vi "S4GUI.vi"() -> ()   [LabVIEW 2018] (continued)
        n871 = call-dynamic "Write State Machine.vi"("error in (no error)"=w1797, "State Machine.lvclass"=w1799, "Device in"=w1801) -> ("error out"=w1782:errorcluster, "Device out"=w1778:refnum<class "Channel.lvclass">)  [unwired: 7 in]
        n872 = call "Write section_name.vi"("error in (no error)"=w1782, "section_name"="CCD_ACS1", "Channel in"=w1778) -> ("error out"=w1783:errorcluster, "Channel out"=w1777:refnum<class "Channel.lvclass">)  [unwired: 7 in]
        n873 = call-dynamic "save config.vi"("error in (no error)"=w1783, "file config"="lastsaved.cfg", "Channel in"=w1777) -> ("error out"=w1781:errorcluster, "Channel out"=w1776:refnum<class "Channel.lvclass">)  [unwired: 7 in]
        n874 = call-dynamic "Write Channel.vi"("error in (no error)"=w1781, "Channel.lvclass"=w1776, "Acquisition in"=w1803) -> ("error out"=w1795:errorcluster, "Acquisition out"=w1794:refnum<class "Acquisition.lvclass">)  [unwired: 7 in]
        n875 = call-dynamic "Write AcquisitionA.vi"("error in (no error)"=w1795, "Acquisition.lvclass"=w1794, "S4ACS_GUI in"=w1805) -> ("error out"=w1793:errorcluster, "S4ACS_GUI out"=w1784:refnum<class "S4GUI.lvclass">)  [unwired: 7 in]
      }
      event "Load Button": Value Change {
        n876 = event-data() -> ()  [unwired: 1 in, 6 out]
        n877 = call <vilib>:"Application Directory.vi"() -> ("Application Directory"=w1819:path)
        n878 = call "File Dialog"("start path"=w1819, "prompt"="Select file...", "button label"="Open", "default name"="lastsaved.cfg", "error in"=w1813, "pattern (all files)"="*.cfg") -> ("selected path"=w1811:path, "cancelled"=w1814:bool, "error out"=→"error out 2":errorcluster)  [unwired: 6 in, 1 out]
        "selected path" <- w1811
        n879 = Path To String(path=w1811) -> (string=w1810:string)
        n880 = Match Pattern(string=w1810, regular expression="SPARC4_GUI\\") -> (after substring=w1808:string)  [unwired: 1 in, 3 out]
        n881 = case shown="False" w1814 {
          tunnel: w1822 -> [w1931 w1933]
          tunnel: [w1847 w1933] -> w1821
          tunnel: [w1845 w1932] -> w1820
          tunnel: w1813 -> [w1844 w1932]
          tunnel: w1808 -> [w1843 _]
          frame False {
            n882 = call-dynamic "Read AcquisitionA.vi"("error in (no error)"=w1844, "S4ACS_GUI in"=w1931) -> ("error out"=w1927:errorcluster, "Acquisition.lvclass"=w1929:refnum<class "Acquisition.lvclass">, "S4ACS_GUI out"=w1930:refnum<class "S4GUI.lvclass">)  [unwired: 7 in]
            n883 = call-dynamic "Read Channel.vi"("error in (no error)"=w1927, "Acquisition in"=w1929) -> ("error out"=w1914:errorcluster, "Channel.lvclass"=w1916:refnum<class "Channel.lvclass">, "Acquisition out"=w1928:refnum<class "Acquisition.lvclass">)  [unwired: 7 in]
            n884 = call "Write section_name.vi"("error in (no error)"=w1914, "section_name"="CCD_ACS1", "Channel in"=w1916) -> ("error out"=w1913:errorcluster, "Channel out"=w1915:refnum<class "Channel.lvclass">)  [unwired: 7 in]
            n885 = call-dynamic "load config.vi"("error in (no error)"=w1913, "cfg file name"=w1843, "Channel in"=w1915) -> ("error out"=w1839:errorcluster, "Channel out"=w1841:refnum<class "Channel.lvclass">)  [unwired: 7 in]
            n886 = call-dynamic "save config.vi"("error in (no error)"=w1839, "file config"="lastsaved.cfg", "Channel in"=w1841) -> ("error out"=w1842:errorcluster, "Channel out"=w1840:refnum<class "Channel.lvclass">)  [unwired: 7 in]
            n887 = call-dynamic "Read State Machine.vi"("error in (no error)"=w1842, "Device in"=w1840) -> ("error out"=w1923:errorcluster, "State Machine.lvclass"=w1925:refnum<class "State Machine.lvclass">, "Device out"=w1926:refnum<class "Channel.lvclass">)  [unwired: 7 in]
            n888 = call-dynamic "Write State.vi"("error in (no error)"=w1923, "State"=60, "State Machine in"=w1925) -> ("error out"=w1922:errorcluster, "State Machine out"=w1924:refnum<class "State Machine.lvclass">)  [unwired: 7 in]
            n889 = call-dynamic "Write State Machine.vi"("error in (no error)"=w1922, "State Machine.lvclass"=w1924, "Device in"=w1926) -> ("error out"=w1919:errorcluster, "Device out"=w1920:refnum<class "Channel.lvclass">)  [unwired: 7 in]
            n890 = call-dynamic "Write Channel.vi"("error in (no error)"=w1919, "Channel.lvclass"=w1920, "Acquisition in"=w1928) -> ("error out"=w1918:errorcluster, "Acquisition out"=w1917:refnum<class "Acquisition.lvclass">)  [unwired: 7 in]
            n891 = call-dynamic "Write AcquisitionA.vi"("error in (no error)"=w1918, "Acquisition.lvclass"=w1917, "S4ACS_GUI in"=w1930) -> ("error out"=w1854:errorcluster, "S4ACS_GUI out"=w1853:refnum<class "S4GUI.lvclass">)  [unwired: 7 in]
            n892 = call "Read AcquisitionB.vi"("error in (no error)"=w1854, "S4ACS_GUI in"=w1853) -> ("error out"=w1896:errorcluster, "Acquisition.lvclass"=w1894:refnum<class "Acquisition.lvclass">, "S4ACS_GUI out"=w1893:refnum<class "S4GUI.lvclass">)  [unwired: 7 in]
            n893 = call-dynamic "Read Channel.vi"("error in (no error)"=w1896, "Acquisition in"=w1894) -> ("error out"=w1909:errorcluster, "Channel.lvclass"=w1907:refnum<class "Channel.lvclass">, "Acquisition out"=w1895:refnum<class "Acquisition.lvclass">)  [unwired: 7 in]
            n894 = call "Write section_name.vi"("error in (no error)"=w1909, "section_name"="CCD_ACS2", "Channel in"=w1907) -> ("error out"=w1910:errorcluster, "Channel out"=w1908:refnum<class "Channel.lvclass">)  [unwired: 7 in]
            n895 = call-dynamic "load config.vi"("error in (no error)"=w1910, "cfg file name"=w1843, "Channel in"=w1908) -> ("error out"=w1836:errorcluster, "Channel out"=w1834:refnum<class "Channel.lvclass">)  [unwired: 7 in]
            n896 = call-dynamic "save config.vi"("error in (no error)"=w1836, "file config"="lastsaved.cfg", "Channel in"=w1834) -> ("error out"=w1835:errorcluster, "Channel out"=w1833:refnum<class "Channel.lvclass">)  [unwired: 7 in]
            n897 = call-dynamic "Read State Machine.vi"("error in (no error)"=w1835, "Device in"=w1833) -> ("error out"=w1900:errorcluster, "State Machine.lvclass"=w1898:refnum<class "State Machine.lvclass">, "Device out"=w1897:refnum<class "Channel.lvclass">)  [unwired: 7 in]
            n898 = call-dynamic "Write State.vi"("error in (no error)"=w1900, "State"=60, "State Machine in"=w1898) -> ("error out"=w1901:errorcluster, "State Machine out"=w1899:refnum<class "State Machine.lvclass">)  [unwired: 7 in]
            n899 = call-dynamic "Write State Machine.vi"("error in (no error)"=w1901, "State Machine.lvclass"=w1899, "Device in"=w1897) -> ("error out"=w1904:errorcluster, "Device out"=w1903:refnum<class "Channel.lvclass">)  [unwired: 7 in]
            n900 = call-dynamic "Write Channel.vi"("error in (no error)"=w1904, "Channel.lvclass"=w1903, "Acquisition in"=w1895) -> ("error out"=w1905:errorcluster, "Acquisition out"=w1906:refnum<class "Acquisition.lvclass">)  [unwired: 7 in]
            n901 = call "Write AcquisitionB.vi"("error in (no error)"=w1905, "Acquisition.lvclass"=w1906, "S4ACS_GUI in"=w1893) -> ("error out"=w1852:errorcluster, "S4ACS_GUI out"=w1851:refnum<class "S4GUI.lvclass">)  [unwired: 7 in]
            n902 = call-dynamic "Read AcquisitionC.vi"("error in (no error)"=w1852, "S4ACS_GUI in"=w1851) -> ("error out"=w1889:errorcluster, "Acquisition.lvclass"=w1891:refnum<class "Acquisition.lvclass">, "S4ACS_GUI out"=w1892:refnum<class "S4GUI.lvclass">)  [unwired: 7 in]
            n903 = call-dynamic "Read Channel.vi"("error in (no error)"=w1889, "Acquisition in"=w1891) -> ("error out"=w1876:errorcluster, "Channel.lvclass"=w1878:refnum<class "Channel.lvclass">, "Acquisition out"=w1890:refnum<class "Acquisition.lvclass">)  [unwired: 7 in]
            n904 = call "Write section_name.vi"("error in (no error)"=w1876, "section_name"="CCD_ACS3", "Channel in"=w1878) -> ("error out"=w1875:errorcluster, "Channel out"=w1877:refnum<class "Channel.lvclass">)  [unwired: 7 in]
            n905 = call-dynamic "load config.vi"("error in (no error)"=w1875, "cfg file name"=w1843, "Channel in"=w1877) -> ("error out"=w1831:errorcluster, "Channel out"=w1829:refnum<class "Channel.lvclass">)  [unwired: 7 in]
            n906 = call-dynamic "save config.vi"("error in (no error)"=w1831, "file config"="lastsaved.cfg", "Channel in"=w1829) -> ("error out"=w1830:errorcluster, "Channel out"=w1828:refnum<class "Channel.lvclass">)  [unwired: 7 in]
            n907 = call-dynamic "Read State Machine.vi"("error in (no error)"=w1830, "Device in"=w1828) -> ("error out"=w1885:errorcluster, "State Machine.lvclass"=w1887:refnum<class "State Machine.lvclass">, "Device out"=w1888:refnum<class "Channel.lvclass">)  [unwired: 7 in]
            n908 = call-dynamic "Write State.vi"("error in (no error)"=w1885, "State"=60, "State Machine in"=w1887) -> ("error out"=w1884:errorcluster, "State Machine out"=w1886:refnum<class "State Machine.lvclass">)  [unwired: 7 in]
            n909 = call-dynamic "Write State Machine.vi"("error in (no error)"=w1884, "State Machine.lvclass"=w1886, "Device in"=w1888) -> ("error out"=w1881:errorcluster, "Device out"=w1882:refnum<class "Channel.lvclass">)  [unwired: 7 in]
            n910 = call-dynamic "Write Channel.vi"("error in (no error)"=w1881, "Channel.lvclass"=w1882, "Acquisition in"=w1890) -> ("error out"=w1880:errorcluster, "Acquisition out"=w1879:refnum<class "Acquisition.lvclass">)  [unwired: 7 in]
            n911 = call-dynamic "Write AcquisitionC.vi"("error in (no error)"=w1880, "Acquisition.lvclass"=w1879, "S4ACS_GUI in"=w1892) -> ("error out"=w1850:errorcluster, "S4ACS_GUI out"=w1849:refnum<class "S4GUI.lvclass">)  [unwired: 7 in]
            n912 = call-dynamic "Read AcquisitionD.vi"("error in (no error)"=w1850, "S4ACS_GUI in"=w1849) -> ("error out"=w1858:errorcluster, "Acquisition.lvclass"=w1856:refnum<class "Acquisition.lvclass">, "S4ACS_GUI out"=w1855:refnum<class "S4GUI.lvclass">)  [unwired: 7 in]
            n913 = call-dynamic "Read Channel.vi"("error in (no error)"=w1858, "Acquisition in"=w1856) -> ("error out"=w1871:errorcluster, "Channel.lvclass"=w1869:refnum<class "Channel.lvclass">, "Acquisition out"=w1857:refnum<class "Acquisition.lvclass">)  [unwired: 7 in]
            n914 = call "Write section_name.vi"("error in (no error)"=w1871, "section_name"="CCD_ACS4", "Channel in"=w1869) -> ("error out"=w1872:errorcluster, "Channel out"=w1870:refnum<class "Channel.lvclass">)  [unwired: 7 in]
            n915 = call-dynamic "load config.vi"("error in (no error)"=w1872, "cfg file name"=w1843, "Channel in"=w1870) -> ("error out"=w1827:errorcluster, "Channel out"=w1825:refnum<class "Channel.lvclass">)  [unwired: 7 in]
            n916 = call-dynamic "save config.vi"("error in (no error)"=w1827, "file config"="lastsaved.cfg", "Channel in"=w1825) -> ("error out"=w1826:errorcluster, "Channel out"=w1824:refnum<class "Channel.lvclass">)  [unwired: 7 in]
            n917 = call-dynamic "Read State Machine.vi"("error in (no error)"=w1826, "Device in"=w1824) -> ("error out"=w1862:errorcluster, "State Machine.lvclass"=w1860:refnum<class "State Machine.lvclass">, "Device out"=w1859:refnum<class "Channel.lvclass">)  [unwired: 7 in]
            n918 = call-dynamic "Write State.vi"("error in (no error)"=w1862, "State"=60, "State Machine in"=w1860) -> ("error out"=w1863:errorcluster, "State Machine out"=w1861:refnum<class "State Machine.lvclass">)  [unwired: 7 in]
            n919 = call-dynamic "Write State Machine.vi"("error in (no error)"=w1863, "State Machine.lvclass"=w1861, "Device in"=w1859) -> ("error out"=w1866:errorcluster, "Device out"=w1865:refnum<class "Channel.lvclass">)  [unwired: 7 in]
            n920 = call-dynamic "Write Channel.vi"("error in (no error)"=w1866, "Channel.lvclass"=w1865, "Acquisition in"=w1857) -> ("error out"=w1867:errorcluster, "Acquisition out"=w1868:refnum<class "Acquisition.lvclass">)  [unwired: 7 in]
            n921 = call-dynamic "Write AcquisitionD.vi"("error in (no error)"=w1867, "Acquisition.lvclass"=w1868, "S4ACS_GUI in"=w1855) -> ("error out"=w1846:errorcluster, "S4ACS_GUI out"=w1848:refnum<class "S4GUI.lvclass">)  [unwired: 7 in]
            n922 = call "Write cfg file.vi"("error in (no error)"=w1846, "cfg file"=w1843, "S4ACS_GUI in"=w1848) -> ("error out"=w1845:errorcluster, "S4ACS_GUI out"=w1847:refnum<class "S4GUI.lvclass">)  [unwired: 7 in]
          }
          frame True {
          }
        }
      }
      event "Save As Button": Value Change {
        n923 = event-data() -> ()  [unwired: 1 in, 6 out]
        n924 = call <vilib>:"Application Directory.vi"() -> ("Application Directory"=w1945:path)
        n925 = call "File Dialog2"("start path"=w1945, "prompt"="Select file...", "button label"="Save", "default name"="lastsaved.cfg", "error in"=w1939, "pattern (all files)"="*.cfg") -> ("selected path"=w1937:path, "cancelled"=w1940:bool, "error out"=→"error out 3":errorcluster)  [unwired: 6 in, 1 out]
        n926 = Path To String(path=w1937) -> (string=w1936:string)
        n927 = Match Pattern(string=w1936, regular expression="SPARC4_GUI\\") -> (after substring=w1934:string)  [unwired: 1 in, 3 out]
        n928 = case shown="False" w1940 {
          tunnel: w1948 -> [w2013 w2015]
          tunnel: [w1961 w2015] -> w1947
          tunnel: [w1959 w2014] -> w1946
          tunnel: w1939 -> [w1958 w2014]
          tunnel: w1934 -> [w1957 _]
          frame False {
            n929 = call-dynamic "Read AcquisitionA.vi"("error in (no error)"=w1958, "S4ACS_GUI in"=w2013) -> ("error out"=w2009:errorcluster, "Acquisition.lvclass"=w2011:refnum<class "Acquisition.lvclass">, "S4ACS_GUI out"=w2012:refnum<class "S4GUI.lvclass">)  [unwired: 7 in]
            n930 = call-dynamic "Read Channel.vi"("error in (no error)"=w2009, "Acquisition in"=w2011) -> ("error out"=w2004:errorcluster, "Channel.lvclass"=w2006:refnum<class "Channel.lvclass">, "Acquisition out"=w2010:refnum<class "Acquisition.lvclass">)  [unwired: 7 in]
            n931 = call "Write section_name.vi"("error in (no error)"=w2004, "section_name"="CCD_ACS1", "Channel in"=w2006) -> ("error out"=w2003:errorcluster, "Channel out"=w2005:refnum<class "Channel.lvclass">)  [unwired: 7 in]
            n932 = call-dynamic "save config.vi"("error in (no error)"=w2003, "file config"=w1957, "Channel in"=w2005) -> ("error out"=w1955:errorcluster, "Channel out"=w1956:refnum<class "Channel.lvclass">)  [unwired: 7 in]
            n933 = call-dynamic "Write Channel.vi"("error in (no error)"=w1955, "Channel.lvclass"=w1956, "Acquisition in"=w2010) -> ("error out"=w2008:errorcluster, "Acquisition out"=w2007:refnum<class "Acquisition.lvclass">)  [unwired: 7 in]
            n934 = call-dynamic "Write AcquisitionA.vi"("error in (no error)"=w2008, "Acquisition.lvclass"=w2007, "S4ACS_GUI in"=w2012) -> ("error out"=w1968:errorcluster, "S4ACS_GUI out"=w1967:refnum<class "S4GUI.lvclass">)  [unwired: 7 in]
            n935 = call "Read AcquisitionB.vi"("error in (no error)"=w1968, "S4ACS_GUI in"=w1967) -> ("error out"=w1994:errorcluster, "Acquisition.lvclass"=w1992:refnum<class "Acquisition.lvclass">, "S4ACS_GUI out"=w1991:refnum<class "S4GUI.lvclass">)  [unwired: 7 in]
            n936 = call-dynamic "Read Channel.vi"("error in (no error)"=w1994, "Acquisition in"=w1992) -> ("error out"=w1999:errorcluster, "Channel.lvclass"=w1997:refnum<class "Channel.lvclass">, "Acquisition out"=w1993:refnum<class "Acquisition.lvclass">)  [unwired: 7 in]
            n937 = call "Write section_name.vi"("error in (no error)"=w1999, "section_name"="CCD_ACS2", "Channel in"=w1997) -> ("error out"=w2000:errorcluster, "Channel out"=w1998:refnum<class "Channel.lvclass">)  [unwired: 7 in]
            n938 = call-dynamic "save config.vi"("error in (no error)"=w2000, "file config"=w1957, "Channel in"=w1998) -> ("error out"=w1949:errorcluster, "Channel out"=w1950:refnum<class "Channel.lvclass">)  [unwired: 7 in]
            n939 = call-dynamic "Write Channel.vi"("error in (no error)"=w1949, "Channel.lvclass"=w1950, "Acquisition in"=w1993) -> ("error out"=w1995:errorcluster, "Acquisition out"=w1996:refnum<class "Acquisition.lvclass">)  [unwired: 7 in]
            n940 = call "Write AcquisitionB.vi"("error in (no error)"=w1995, "Acquisition.lvclass"=w1996, "S4ACS_GUI in"=w1991) -> ("error out"=w1966:errorcluster, "S4ACS_GUI out"=w1965:refnum<class "S4GUI.lvclass">)  [unwired: 7 in]
            n941 = call-dynamic "Read AcquisitionC.vi"("error in (no error)"=w1966, "S4ACS_GUI in"=w1965) -> ("error out"=w1987:errorcluster, "Acquisition.lvclass"=w1989:refnum<class "Acquisition.lvclass">, "S4ACS_GUI out"=w1990:refnum<class "S4GUI.lvclass">)  [unwired: 7 in]
            n942 = call-dynamic "Read Channel.vi"("error in (no error)"=w1987, "Acquisition in"=w1989) -> ("error out"=w1982:errorcluster, "Channel.lvclass"=w1984:refnum<class "Channel.lvclass">, "Acquisition out"=w1988:refnum<class "Acquisition.lvclass">)  [unwired: 7 in]
            n943 = call "Write section_name.vi"("error in (no error)"=w1982, "section_name"="CCD_ACS3", "Channel in"=w1984) -> ("error out"=w1981:errorcluster, "Channel out"=w1983:refnum<class "Channel.lvclass">)  [unwired: 7 in]
            n944 = call-dynamic "save config.vi"("error in (no error)"=w1981, "file config"=w1957, "Channel in"=w1983) -> ("error out"=w1951:errorcluster, "Channel out"=w1952:refnum<class "Channel.lvclass">)  [unwired: 7 in]
            n945 = call-dynamic "Write Channel.vi"("error in (no error)"=w1951, "Channel.lvclass"=w1952, "Acquisition in"=w1988) -> ("error out"=w1986:errorcluster, "Acquisition out"=w1985:refnum<class "Acquisition.lvclass">)  [unwired: 7 in]
            n946 = call-dynamic "Write AcquisitionC.vi"("error in (no error)"=w1986, "Acquisition.lvclass"=w1985, "S4ACS_GUI in"=w1990) -> ("error out"=w1964:errorcluster, "S4ACS_GUI out"=w1963:refnum<class "S4GUI.lvclass">)  [unwired: 7 in]
            n947 = call-dynamic "Read AcquisitionD.vi"("error in (no error)"=w1964, "S4ACS_GUI in"=w1963) -> ("error out"=w1972:errorcluster, "Acquisition.lvclass"=w1970:refnum<class "Acquisition.lvclass">, "S4ACS_GUI out"=w1969:refnum<class "S4GUI.lvclass">)  [unwired: 7 in]
            n948 = call-dynamic "Read Channel.vi"("error in (no error)"=w1972, "Acquisition in"=w1970) -> ("error out"=w1977:errorcluster, "Channel.lvclass"=w1975:refnum<class "Channel.lvclass">, "Acquisition out"=w1971:refnum<class "Acquisition.lvclass">)  [unwired: 7 in]
            n949 = call "Write section_name.vi"("error in (no error)"=w1977, "section_name"="CCD_ACS4", "Channel in"=w1975) -> ("error out"=w1978:errorcluster, "Channel out"=w1976:refnum<class "Channel.lvclass">)  [unwired: 7 in]
            n950 = call-dynamic "save config.vi"("error in (no error)"=w1978, "file config"=w1957, "Channel in"=w1976) -> ("error out"=w1953:errorcluster, "Channel out"=w1954:refnum<class "Channel.lvclass">)  [unwired: 7 in]
            n951 = call-dynamic "Write Channel.vi"("error in (no error)"=w1953, "Channel.lvclass"=w1954, "Acquisition in"=w1971) -> ("error out"=w1973:errorcluster, "Acquisition out"=w1974:refnum<class "Acquisition.lvclass">)  [unwired: 7 in]
            n952 = call-dynamic "Write AcquisitionD.vi"("error in (no error)"=w1973, "Acquisition.lvclass"=w1974, "S4ACS_GUI in"=w1969) -> ("error out"=w1960:errorcluster, "S4ACS_GUI out"=w1962:refnum<class "S4GUI.lvclass">)  [unwired: 7 in]
            n953 = call "Write cfg file.vi"("error in (no error)"=w1960, "cfg file"=w1957, "S4ACS_GUI in"=w1962) -> ("error out"=w1959:errorcluster, "S4ACS_GUI out"=w1961:refnum<class "S4GUI.lvclass">)  [unwired: 7 in]
          }
          frame True {
          }
        }
      }
      event "Load Default Button": Value Change {
        w2036 = "default.cfg" ("cfg file name")
        n954 = event-data() -> ()  [unwired: 1 in, 6 out]
        n955 = call-dynamic "Read AcquisitionA.vi"("error in (no error)"=w2126, "S4ACS_GUI in"=w2127) -> ("error out"=w2122:errorcluster, "Acquisition.lvclass"=w2124:refnum<class "Acquisition.lvclass">, "S4ACS_GUI out"=w2125:refnum<class "S4GUI.lvclass">)  [unwired: 7 in]
        n956 = call-dynamic "Read Channel.vi"("error in (no error)"=w2122, "Acquisition in"=w2124) -> ("error out"=w2109:errorcluster, "Channel.lvclass"=w2111:refnum<class "Channel.lvclass">, "Acquisition out"=w2123:refnum<class "Acquisition.lvclass">)  [unwired: 7 in]
        n957 = call "Write section_name.vi"("error in (no error)"=w2109, "section_name"="CCD_ACS1", "Channel in"=w2111) -> ("error out"=w2108:errorcluster, "Channel out"=w2110:refnum<class "Channel.lvclass">)  [unwired: 7 in]
        n958 = call-dynamic "load config.vi"("error in (no error)"=w2108, "cfg file name"=w2036, "Channel in"=w2110) -> ("error out"=w2033:errorcluster, "Channel out"=w2035:refnum<class "Channel.lvclass">)  [unwired: 7 in]
        n959 = call-dynamic "save config.vi"("error in (no error)"=w2033, "file config"="lastsaved.cfg", "Channel in"=w2035) -> ("error out"=w2032:errorcluster, "Channel out"=w2034:refnum<class "Channel.lvclass">)  [unwired: 7 in]
        n960 = call-dynamic "Read State Machine.vi"("error in (no error)"=w2032, "Device in"=w2034) -> ("error out"=w2118:errorcluster, "State Machine.lvclass"=w2120:refnum<class "State Machine.lvclass">, "Device out"=w2121:refnum<class "Channel.lvclass">)  [unwired: 7 in]
        n961 = call-dynamic "Write State.vi"("error in (no error)"=w2118, "State"=60, "State Machine in"=w2120) -> ("error out"=w2117:errorcluster, "State Machine out"=w2119:refnum<class "State Machine.lvclass">)  [unwired: 7 in]
        n962 = call-dynamic "Write State Machine.vi"("error in (no error)"=w2117, "State Machine.lvclass"=w2119, "Device in"=w2121) -> ("error out"=w2114:errorcluster, "Device out"=w2115:refnum<class "Channel.lvclass">)  [unwired: 7 in]
        n963 = call-dynamic "Write Channel.vi"("error in (no error)"=w2114, "Channel.lvclass"=w2115, "Acquisition in"=w2123) -> ("error out"=w2113:errorcluster, "Acquisition out"=w2112:refnum<class "Acquisition.lvclass">)  [unwired: 7 in]
        n964 = call-dynamic "Write AcquisitionA.vi"("error in (no error)"=w2113, "Acquisition.lvclass"=w2112, "S4ACS_GUI in"=w2125) -> ("error out"=w2046:errorcluster, "S4ACS_GUI out"=w2045:refnum<class "S4GUI.lvclass">)  [unwired: 7 in]
        n965 = call "Read AcquisitionB.vi"("error in (no error)"=w2046, "S4ACS_GUI in"=w2045) -> ("error out"=w2090:errorcluster, "Acquisition.lvclass"=w2088:refnum<class "Acquisition.lvclass">, "S4ACS_GUI out"=w2087:refnum<class "S4GUI.lvclass">)  [unwired: 7 in]
        n966 = call-dynamic "Read Channel.vi"("error in (no error)"=w2090, "Acquisition in"=w2088) -> ("error out"=w2104:errorcluster, "Channel.lvclass"=w2102:refnum<class "Channel.lvclass">, "Acquisition out"=w2089:refnum<class "Acquisition.lvclass">)  [unwired: 7 in]
        n967 = call "Write section_name.vi"("error in (no error)"=w2104, "section_name"="CCD_ACS2", "Channel in"=w2102) -> ("error out"=w2105:errorcluster, "Channel out"=w2103:refnum<class "Channel.lvclass">)  [unwired: 7 in]
        n968 = call-dynamic "load config.vi"("error in (no error)"=w2105, "cfg file name"="default.cfg", "Channel in"=w2103) -> ("error out"=w2029:errorcluster, "Channel out"=w2027:refnum<class "Channel.lvclass">)  [unwired: 7 in]
        n969 = call-dynamic "save config.vi"("error in (no error)"=w2029, "file config"="lastsaved.cfg", "Channel in"=w2027) -> ("error out"=w2028:errorcluster, "Channel out"=w2026:refnum<class "Channel.lvclass">)  [unwired: 7 in]
        n970 = call-dynamic "Read State Machine.vi"("error in (no error)"=w2028, "Device in"=w2026) -> ("error out"=w2094:errorcluster, "State Machine.lvclass"=w2092:refnum<class "State Machine.lvclass">, "Device out"=w2091:refnum<class "Channel.lvclass">)  [unwired: 7 in]
        n971 = call-dynamic "Write State.vi"("error in (no error)"=w2094, "State"=60, "State Machine in"=w2092) -> ("error out"=w2095:errorcluster, "State Machine out"=w2093:refnum<class "State Machine.lvclass">)  [unwired: 7 in]
        n972 = call-dynamic "Write State Machine.vi"("error in (no error)"=w2095, "State Machine.lvclass"=w2093, "Device in"=w2091) -> ("error out"=w2098:errorcluster, "Device out"=w2097:refnum<class "Channel.lvclass">)  [unwired: 7 in]
        n973 = call-dynamic "Write Channel.vi"("error in (no error)"=w2098, "Channel.lvclass"=w2097, "Acquisition in"=w2089) -> ("error out"=w2099:errorcluster, "Acquisition out"=w2100:refnum<class "Acquisition.lvclass">)  [unwired: 7 in]
        n974 = call "Write AcquisitionB.vi"("error in (no error)"=w2099, "Acquisition.lvclass"=w2100, "S4ACS_GUI in"=w2087) -> ("error out"=w2044:errorcluster, "S4ACS_GUI out"=w2043:refnum<class "S4GUI.lvclass">)  [unwired: 7 in]
        n975 = call-dynamic "Read AcquisitionC.vi"("error in (no error)"=w2044, "S4ACS_GUI in"=w2043) -> ("error out"=w2083:errorcluster, "Acquisition.lvclass"=w2085:refnum<class "Acquisition.lvclass">, "S4ACS_GUI out"=w2086:refnum<class "S4GUI.lvclass">)  [unwired: 7 in]
        n976 = call-dynamic "Read Channel.vi"("error in (no error)"=w2083, "Acquisition in"=w2085) -> ("error out"=w2069:errorcluster, "Channel.lvclass"=w2071:refnum<class "Channel.lvclass">, "Acquisition out"=w2084:refnum<class "Acquisition.lvclass">)  [unwired: 7 in]
        n977 = call "Write section_name.vi"("error in (no error)"=w2069, "section_name"="CCD_ACS3", "Channel in"=w2071) -> ("error out"=w2068:errorcluster, "Channel out"=w2070:refnum<class "Channel.lvclass">)  [unwired: 7 in]
        n978 = call-dynamic "load config.vi"("error in (no error)"=w2068, "cfg file name"="default.cfg", "Channel in"=w2070) -> ("error out"=w2023:errorcluster, "Channel out"=w2024:refnum<class "Channel.lvclass">)  [unwired: 7 in]
        n979 = call-dynamic "save config.vi"("error in (no error)"=w2023, "file config"="lastsaved.cfg", "Channel in"=w2024) -> ("error out"=w2021:errorcluster, "Channel out"=w2022:refnum<class "Channel.lvclass">)  [unwired: 7 in]
        n980 = call-dynamic "Read State Machine.vi"("error in (no error)"=w2021, "Device in"=w2022) -> ("error out"=w2079:errorcluster, "State Machine.lvclass"=w2081:refnum<class "State Machine.lvclass">, "Device out"=w2082:refnum<class "Channel.lvclass">)  [unwired: 7 in]
        n981 = call-dynamic "Write State.vi"("error in (no error)"=w2079, "State"=60, "State Machine in"=w2081) -> ("error out"=w2078:errorcluster, "State Machine out"=w2080:refnum<class "State Machine.lvclass">)  [unwired: 7 in]
        n982 = call-dynamic "Write State Machine.vi"("error in (no error)"=w2078, "State Machine.lvclass"=w2080, "Device in"=w2082) -> ("error out"=w2075:errorcluster, "Device out"=w2076:refnum<class "Channel.lvclass">)  [unwired: 7 in]
        n983 = call-dynamic "Write Channel.vi"("error in (no error)"=w2075, "Channel.lvclass"=w2076, "Acquisition in"=w2084) -> ("error out"=w2074:errorcluster, "Acquisition out"=w2073:refnum<class "Acquisition.lvclass">)  [unwired: 7 in]
        n984 = call-dynamic "Write AcquisitionC.vi"("error in (no error)"=w2074, "Acquisition.lvclass"=w2073, "S4ACS_GUI in"=w2086) -> ("error out"=w2042:errorcluster, "S4ACS_GUI out"=w2041:refnum<class "S4GUI.lvclass">)  [unwired: 7 in]
        n985 = call-dynamic "Read AcquisitionD.vi"("error in (no error)"=w2042, "S4ACS_GUI in"=w2041) -> ("error out"=w2050:errorcluster, "Acquisition.lvclass"=w2048:refnum<class "Acquisition.lvclass">, "S4ACS_GUI out"=w2047:refnum<class "S4GUI.lvclass">)  [unwired: 7 in]
        n986 = call-dynamic "Read Channel.vi"("error in (no error)"=w2050, "Acquisition in"=w2048) -> ("error out"=w2064:errorcluster, "Channel.lvclass"=w2062:refnum<class "Channel.lvclass">, "Acquisition out"=w2049:refnum<class "Acquisition.lvclass">)  [unwired: 7 in]
        n987 = call "Write section_name.vi"("error in (no error)"=w2064, "section_name"="CCD_ACS4", "Channel in"=w2062) -> ("error out"=w2065:errorcluster, "Channel out"=w2063:refnum<class "Channel.lvclass">)  [unwired: 7 in]
        n988 = call-dynamic "load config.vi"("error in (no error)"=w2065, "cfg file name"="default.cfg", "Channel in"=w2063) -> ("error out"=w2019:errorcluster, "Channel out"=w2018:refnum<class "Channel.lvclass">)  [unwired: 7 in]
        n989 = call-dynamic "save config.vi"("error in (no error)"=w2019, "file config"="lastsaved.cfg", "Channel in"=w2018) -> ("error out"=w2016:errorcluster, "Channel out"=w2017:refnum<class "Channel.lvclass">)  [unwired: 7 in]
        n990 = call-dynamic "Read State Machine.vi"("error in (no error)"=w2016, "Device in"=w2017) -> ("error out"=w2054:errorcluster, "State Machine.lvclass"=w2052:refnum<class "State Machine.lvclass">, "Device out"=w2051:refnum<class "Channel.lvclass">)  [unwired: 7 in]
        n991 = call-dynamic "Write State.vi"("error in (no error)"=w2054, "State"=60, "State Machine in"=w2052) -> ("error out"=w2055:errorcluster, "State Machine out"=w2053:refnum<class "State Machine.lvclass">)  [unwired: 7 in]
        n992 = call-dynamic "Write State Machine.vi"("error in (no error)"=w2055, "State Machine.lvclass"=w2053, "Device in"=w2051) -> ("error out"=w2058:errorcluster, "Device out"=w2057:refnum<class "Channel.lvclass">)  [unwired: 7 in]
        n993 = call-dynamic "Write Channel.vi"("error in (no error)"=w2058, "Channel.lvclass"=w2057, "Acquisition in"=w2049) -> ("error out"=w2059:errorcluster, "Acquisition out"=w2060:refnum<class "Acquisition.lvclass">)  [unwired: 7 in]
        n994 = call-dynamic "Write AcquisitionD.vi"("error in (no error)"=w2059, "Acquisition.lvclass"=w2060, "S4ACS_GUI in"=w2047) -> ("error out"=w2038:errorcluster, "S4ACS_GUI out"=w2040:refnum<class "S4GUI.lvclass">)  [unwired: 7 in]
        n995 = call "Write cfg file.vi"("error in (no error)"=w2038, "cfg file"=w2036, "S4ACS_GUI in"=w2040) -> ("error out"=w2037:errorcluster, "S4ACS_GUI out"=w2039:refnum<class "S4GUI.lvclass">)  [unwired: 7 in]
      }
      event "Restore Default ch2": Value Change {
        n996 = event-data() -> ()  [unwired: 1 in, 6 out]
        n997 = call "Read AcquisitionB.vi"("error in (no error)"=w2158, "S4ACS_GUI in"=w2159) -> ("error out"=w2154:errorcluster, "Acquisition.lvclass"=w2156:refnum<class "Acquisition.lvclass">, "S4ACS_GUI out"=w2157:refnum<class "S4GUI.lvclass">)  [unwired: 7 in]
        n998 = call-dynamic "Read Channel.vi"("error in (no error)"=w2154, "Acquisition in"=w2156) -> ("error out"=w2141:errorcluster, "Channel.lvclass"=w2143:refnum<class "Channel.lvclass">, "Acquisition out"=w2155:refnum<class "Acquisition.lvclass">)  [unwired: 7 in]
        n999 = call "Write section_name.vi"("error in (no error)"=w2141, "section_name"="CCD_ACS2", "Channel in"=w2143) -> ("error out"=w2140:errorcluster, "Channel out"=w2142:refnum<class "Channel.lvclass">)  [unwired: 7 in]
        n1000 = call-dynamic "load config.vi"("error in (no error)"=w2140, "cfg file name"="default.cfg", "Channel in"=w2142) -> ("error out"=w2138:errorcluster, "Channel out"=w2139:refnum<class "Channel.lvclass">)  [unwired: 7 in]
        n1001 = call-dynamic "Read State Machine.vi"("error in (no error)"=w2138, "Device in"=w2139) -> ("error out"=w2150:errorcluster, "State Machine.lvclass"=w2152:refnum<class "State Machine.lvclass">, "Device out"=w2153:refnum<class "Channel.lvclass">)  [unwired: 7 in]
        n1002 = call-dynamic "Write State.vi"("error in (no error)"=w2150, "State"=60, "State Machine in"=w2152) -> ("error out"=w2149:errorcluster, "State Machine out"=w2151:refnum<class "State Machine.lvclass">)  [unwired: 7 in]
        n1003 = call-dynamic "Write State Machine.vi"("error in (no error)"=w2149, "State Machine.lvclass"=w2151, "Device in"=w2153) -> ("error out"=w2134:errorcluster, "Device out"=w2131:refnum<class "Channel.lvclass">)  [unwired: 7 in]
        n1004 = call "Write section_name.vi"("error in (no error)"=w2134, "section_name"="CCD_ACS2", "Channel in"=w2131) -> ("error out"=w2135:errorcluster, "Channel out"=w2130:refnum<class "Channel.lvclass">)  [unwired: 7 in]
        n1005 = call-dynamic "save config.vi"("error in (no error)"=w2135, "file config"="lastsaved.cfg", "Channel in"=w2130) -> ("error out"=w2133:errorcluster, "Channel out"=w2129:refnum<class "Channel.lvclass">)  [unwired: 7 in]
        n1006 = call-dynamic "Write Channel.vi"("error in (no error)"=w2133, "Channel.lvclass"=w2129, "Acquisition in"=w2155) -> ("error out"=w2147:errorcluster, "Acquisition out"=w2146:refnum<class "Acquisition.lvclass">)  [unwired: 7 in]
        n1007 = call "Write AcquisitionB.vi"("error in (no error)"=w2147, "Acquisition.lvclass"=w2146, "S4ACS_GUI in"=w2157) -> ("error out"=w2145:errorcluster, "S4ACS_GUI out"=w2136:refnum<class "S4GUI.lvclass">)  [unwired: 7 in]
      }
      event "Restore Default ch3": Value Change {
        n1008 = event-data() -> ()  [unwired: 1 in, 6 out]
        n1009 = call-dynamic "Read AcquisitionC.vi"("error in (no error)"=w2190, "S4ACS_GUI in"=w2191) -> ("error out"=w2186:errorcluster, "Acquisition.lvclass"=w2188:refnum<class "Acquisition.lvclass">, "S4ACS_GUI out"=w2189:refnum<class "S4GUI.lvclass">)  [unwired: 7 in]
        n1010 = call-dynamic "Read Channel.vi"("error in (no error)"=w2186, "Acquisition in"=w2188) -> ("error out"=w2173:errorcluster, "Channel.lvclass"=w2175:refnum<class "Channel.lvclass">, "Acquisition out"=w2187:refnum<class "Acquisition.lvclass">)  [unwired: 7 in]
        n1011 = call "Write section_name.vi"("error in (no error)"=w2173, "section_name"="CCD_ACS3", "Channel in"=w2175) -> ("error out"=w2172:errorcluster, "Channel out"=w2174:refnum<class "Channel.lvclass">)  [unwired: 7 in]
        n1012 = call-dynamic "load config.vi"("error in (no error)"=w2172, "cfg file name"="default.cfg", "Channel in"=w2174) -> ("error out"=w2170:errorcluster, "Channel out"=w2171:refnum<class "Channel.lvclass">)  [unwired: 7 in]
        n1013 = call-dynamic "Read State Machine.vi"("error in (no error)"=w2170, "Device in"=w2171) -> ("error out"=w2182:errorcluster, "State Machine.lvclass"=w2184:refnum<class "State Machine.lvclass">, "Device out"=w2185:refnum<class "Channel.lvclass">)  [unwired: 7 in]
        n1014 = call-dynamic "Write State.vi"("error in (no error)"=w2182, "State"=60, "State Machine in"=w2184) -> ("error out"=w2181:errorcluster, "State Machine out"=w2183:refnum<class "State Machine.lvclass">)  [unwired: 7 in]
        n1015 = call-dynamic "Write State Machine.vi"("error in (no error)"=w2181, "State Machine.lvclass"=w2183, "Device in"=w2185) -> ("error out"=w2161:errorcluster, "Device out"=w2163:refnum<class "Channel.lvclass">)  [unwired: 7 in]
        n1016 = call "Write section_name.vi"("error in (no error)"=w2161, "section_name"="CCD_ACS3", "Channel in"=w2163) -> ("error out"=w2167:errorcluster, "Channel out"=w2162:refnum<class "Channel.lvclass">)  [unwired: 7 in]
        n1017 = call-dynamic "save config.vi"("error in (no error)"=w2167, "file config"="lastsaved.cfg", "Channel in"=w2162) -> ("error out"=w2160:errorcluster, "Channel out"=w2164:refnum<class "Channel.lvclass">)  [unwired: 7 in]
        n1018 = call-dynamic "Write Channel.vi"("error in (no error)"=w2160, "Channel.lvclass"=w2164, "Acquisition in"=w2187) -> ("error out"=w2179:errorcluster, "Acquisition out"=w2178:refnum<class "Acquisition.lvclass">)  [unwired: 7 in]
        n1019 = call-dynamic "Write AcquisitionC.vi"("error in (no error)"=w2179, "Acquisition.lvclass"=w2178, "S4ACS_GUI in"=w2189) -> ("error out"=w2177:errorcluster, "S4ACS_GUI out"=w2168:refnum<class "S4GUI.lvclass">)  [unwired: 7 in]
      }
      event "Restore Default ch4": Value Change {
        n1020 = event-data() -> ()  [unwired: 1 in, 6 out]
        n1021 = call-dynamic "Read AcquisitionD.vi"("error in (no error)"=w2222, "S4ACS_GUI in"=w2223) -> ("error out"=w2218:errorcluster, "Acquisition.lvclass"=w2220:refnum<class "Acquisition.lvclass">, "S4ACS_GUI out"=w2221:refnum<class "S4GUI.lvclass">)  [unwired: 7 in]
        n1022 = call-dynamic "Read Channel.vi"("error in (no error)"=w2218, "Acquisition in"=w2220) -> ("error out"=w2205:errorcluster, "Channel.lvclass"=w2207:refnum<class "Channel.lvclass">, "Acquisition out"=w2219:refnum<class "Acquisition.lvclass">)  [unwired: 7 in]
        n1023 = call "Write section_name.vi"("error in (no error)"=w2205, "section_name"="CCD_ACS4", "Channel in"=w2207) -> ("error out"=w2204:errorcluster, "Channel out"=w2206:refnum<class "Channel.lvclass">)  [unwired: 7 in]
        n1024 = call-dynamic "load config.vi"("error in (no error)"=w2204, "cfg file name"="default.cfg", "Channel in"=w2206) -> ("error out"=w2202:errorcluster, "Channel out"=w2203:refnum<class "Channel.lvclass">)  [unwired: 7 in]
        n1025 = call-dynamic "Read State Machine.vi"("error in (no error)"=w2202, "Device in"=w2203) -> ("error out"=w2214:errorcluster, "State Machine.lvclass"=w2216:refnum<class "State Machine.lvclass">, "Device out"=w2217:refnum<class "Channel.lvclass">)  [unwired: 7 in]
        n1026 = call-dynamic "Write State.vi"("error in (no error)"=w2214, "State"=60, "State Machine in"=w2216) -> ("error out"=w2213:errorcluster, "State Machine out"=w2215:refnum<class "State Machine.lvclass">)  [unwired: 7 in]
        n1027 = call-dynamic "Write State Machine.vi"("error in (no error)"=w2213, "State Machine.lvclass"=w2215, "Device in"=w2217) -> ("error out"=w2193:errorcluster, "Device out"=w2196:refnum<class "Channel.lvclass">)  [unwired: 7 in]
        n1028 = call "Write section_name.vi"("error in (no error)"=w2193, "section_name"="CCD_ACS4", "Channel in"=w2196) -> ("error out"=w2199:errorcluster, "Channel out"=w2195:refnum<class "Channel.lvclass">)  [unwired: 7 in]
        n1029 = call-dynamic "save config.vi"("error in (no error)"=w2199, "file config"="lastsaved.cfg", "Channel in"=w2195) -> ("error out"=w2192:errorcluster, "Channel out"=w2194:refnum<class "Channel.lvclass">)  [unwired: 7 in]
        n1030 = call-dynamic "Write Channel.vi"("error in (no error)"=w2192, "Channel.lvclass"=w2194, "Acquisition in"=w2219) -> ("error out"=w2211:errorcluster, "Acquisition out"=w2210:refnum<class "Acquisition.lvclass">)  [unwired: 7 in]
        n1031 = call-dynamic "Write AcquisitionD.vi"("error in (no error)"=w2211, "Acquisition.lvclass"=w2210, "S4ACS_GUI in"=w2221) -> ("error out"=w2209:errorcluster, "S4ACS_GUI out"=w2200:refnum<class "S4GUI.lvclass">)  [unwired: 7 in]
      }
      event "Copy to Input ch1": Value Change {
        n1032 = event-data() -> ()  [unwired: 1 in, 6 out]
        n1033 = call-dynamic "Read AcquisitionA.vi"("error in (no error)"=w2256, "S4ACS_GUI in"=w2257) -> ("error out"=w2252:errorcluster, "Acquisition.lvclass"=w2255:refnum<class "Acquisition.lvclass">, "S4ACS_GUI out"=w2224:refnum<class "S4GUI.lvclass">)  [unwired: 7 in]
        n1034 = call-dynamic "Read Channel.vi"("error in (no error)"=w2252, "Acquisition in"=w2255) -> ("error out"=w2251:errorcluster, "Channel.lvclass"=w2254:refnum<class "Channel.lvclass">)  [unwired: 7 in, 1 out]
        n1035 = call-dynamic "Read Interface.vi"("error in (no error)"=w2251, "Channel in"=w2254) -> ("error out"=w2250:errorcluster, "Interface.lvclass"=w2253:refnum<class "Interface.lvclass">)  [unwired: 7 in, 1 out]
        n1036 = call-dynamic "Get CCD_Config.vi"("error in (no error)"=w2250, "Interface in"=w2253) -> ("error out"=w2247:errorcluster, "output cluster"=w2246:T24)  [unwired: 7 in, 1 out]
        n1037 = Unbundle By Name(w2246) -> ("INITIAL_LINE"=w2245:u16, "INITIAL_COLUMN"=w2244:u16, "FINAL_LINE"=w2243:u16, "FINAL_COLUMN"=w2242:u16, "VBIN"=w2241:u16, "HBIN"=w2240:u16, "PREAMP"=w2239:u8, "EM_GAIN"=w2238:u16, "READOUT_RATE"=w2237:u8, "SHUTTER_OPENING_TIME"=w2236:u16, "SHUTTER_CLOSING_TIME"=w2235:u16, "VERTICAL_SHIFT_SPEED"=w2234:u8, "READ_MODE"=w2233:u8, "VERTICAL_CLOCK_VOLTAGE"=w2232:u8, "AD_CHANNEL"=w2231:u32, "SHUTTER_MODE"=w2230:u8, "SHUTTER_TTL"=w2229:u8, "TRIGGER_MODE"=w2228:u8, "FRAME_TRANSFER"=w2227:bool, "ACQUISITION_MODE"=w2226:u8, "EM_MODE"=w2225:u8)
        n1038 = local read "Input Cluster"() -> (w2249:T5)
        n1039 = Bundle By Name(cluster=w2249, "Parameters.Image \nInitial Line"=w2245, "Parameters.Image\nInitial Column"=w2244, "Parameters.Image\nFinal Line"=w2243, "Parameters.Image\nFInal Column"=w2242, "Parameters.Vertical\nBinning"=w2241, "Parameters.Horizontal\nBinning"=w2240, "Parameters.Pre-amplification\nGain"=w2239, "Parameters.CCD\nEM Gain"=w2238, "Parameters.Readout\nRate"=w2237, "Parameters.Shutter\nOpenning Time"=w2236, "Parameters.Shutter\nClosing Time"=w2235, "Parameters.Vertical\nShift Speed"=w2234, "Parameters.Read\nMode"=w2233, "Parameters.Vertical\nClock Voltage"=w2232, "Parameters.A/D \nChannel"=w2231, "Parameters.Shutter\nMode"=w2230, "Parameters.Shutter\nTTL"=w2229, "Parameters.Trigger\nMode"=w2228, "Parameters.Frame\nTransfer"=w2227, "Parameters.Acquisition\nMode"=w2226, "Parameters.CCD \nEM Mode"=w2225) -> (w2248:T5)
        n1040 = local write "Input Cluster"(w2248) -> ()
      }
      event "Copy to Input ch2": Value Change {
        n1041 = event-data() -> ()  [unwired: 1 in, 6 out]
        n1042 = call "Read AcquisitionB.vi"("error in (no error)"=w2290, "S4ACS_GUI in"=w2291) -> ("error out"=w2286:errorcluster, "Acquisition.lvclass"=w2289:refnum<class "Acquisition.lvclass">, "S4ACS_GUI out"=w2258:refnum<class "S4GUI.lvclass">)  [unwired: 7 in]
        n1043 = call-dynamic "Read Channel.vi"("error in (no error)"=w2286, "Acquisition in"=w2289) -> ("error out"=w2285:errorcluster, "Channel.lvclass"=w2288:refnum<class "Channel.lvclass">)  [unwired: 7 in, 1 out]
        n1044 = call-dynamic "Read Interface.vi"("error in (no error)"=w2285, "Channel in"=w2288) -> ("error out"=w2284:errorcluster, "Interface.lvclass"=w2287:refnum<class "Interface.lvclass">)  [unwired: 7 in, 1 out]
        n1045 = call-dynamic "Get CCD_Config.vi"("error in (no error)"=w2284, "Interface in"=w2287) -> ("error out"=w2281:errorcluster, "output cluster"=w2280:T24)  [unwired: 7 in, 1 out]
        n1046 = Unbundle By Name(w2280) -> ("INITIAL_LINE"=w2279:u16, "INITIAL_COLUMN"=w2278:u16, "FINAL_LINE"=w2277:u16, "FINAL_COLUMN"=w2276:u16, "VBIN"=w2275:u16, "HBIN"=w2274:u16, "PREAMP"=w2273:u8, "EM_GAIN"=w2272:u16, "READOUT_RATE"=w2271:u8, "SHUTTER_OPENING_TIME"=w2270:u16, "SHUTTER_CLOSING_TIME"=w2269:u16, "VERTICAL_SHIFT_SPEED"=w2268:u8, "READ_MODE"=w2267:u8, "VERTICAL_CLOCK_VOLTAGE"=w2266:u8, "AD_CHANNEL"=w2265:u32, "SHUTTER_MODE"=w2264:u8, "SHUTTER_TTL"=w2263:u8, "TRIGGER_MODE"=w2262:u8, "FRAME_TRANSFER"=w2261:bool, "ACQUISITION_MODE"=w2260:u8, "EM_MODE"=w2259:u8)
        n1047 = local read "Input Cluster"() -> (w2283:T5)
        n1048 = Bundle By Name(cluster=w2283, "Parameters.Image \nInitial Line"=w2279, "Parameters.Image\nInitial Column"=w2278, "Parameters.Image\nFinal Line"=w2277, "Parameters.Image\nFInal Column"=w2276, "Parameters.Vertical\nBinning"=w2275, "Parameters.Horizontal\nBinning"=w2274, "Parameters.Pre-amplification\nGain"=w2273, "Parameters.CCD\nEM Gain"=w2272, "Parameters.Readout\nRate"=w2271, "Parameters.Shutter\nOpenning Time"=w2270, "Parameters.Shutter\nClosing Time"=w2269, "Parameters.Vertical\nShift Speed"=w2268, "Parameters.Read\nMode"=w2267, "Parameters.Vertical\nClock Voltage"=w2266, "Parameters.A/D \nChannel"=w2265, "Parameters.Shutter\nMode"=w2264, "Parameters.Shutter\nTTL"=w2263, "Parameters.Trigger\nMode"=w2262, "Parameters.Frame\nTransfer"=w2261, "Parameters.Acquisition\nMode"=w2260, "Parameters.CCD \nEM Mode"=w2259) -> (w2282:T5)
        n1049 = local write "Input Cluster"(w2282) -> ()
      }
      event "Copy to Input ch3": Value Change {
        n1050 = event-data() -> ()  [unwired: 1 in, 6 out]
        n1051 = call-dynamic "Read AcquisitionC.vi"("error in (no error)"=w2324, "S4ACS_GUI in"=w2325) -> ("error out"=w2320:errorcluster, "Acquisition.lvclass"=w2323:refnum<class "Acquisition.lvclass">, "S4ACS_GUI out"=w2292:refnum<class "S4GUI.lvclass">)  [unwired: 7 in]
        n1052 = call-dynamic "Read Channel.vi"("error in (no error)"=w2320, "Acquisition in"=w2323) -> ("error out"=w2319:errorcluster, "Channel.lvclass"=w2322:refnum<class "Channel.lvclass">)  [unwired: 7 in, 1 out]
        n1053 = call-dynamic "Read Interface.vi"("error in (no error)"=w2319, "Channel in"=w2322) -> ("error out"=w2318:errorcluster, "Interface.lvclass"=w2321:refnum<class "Interface.lvclass">)  [unwired: 7 in, 1 out]
        n1054 = call-dynamic "Get CCD_Config.vi"("error in (no error)"=w2318, "Interface in"=w2321) -> ("error out"=w2315:errorcluster, "output cluster"=w2314:T24)  [unwired: 7 in, 1 out]
        n1055 = Unbundle By Name(w2314) -> ("INITIAL_LINE"=w2313:u16, "INITIAL_COLUMN"=w2312:u16, "FINAL_LINE"=w2311:u16, "FINAL_COLUMN"=w2310:u16, "VBIN"=w2309:u16, "HBIN"=w2308:u16, "PREAMP"=w2307:u8, "EM_GAIN"=w2306:u16, "READOUT_RATE"=w2305:u8, "SHUTTER_OPENING_TIME"=w2304:u16, "SHUTTER_CLOSING_TIME"=w2303:u16, "VERTICAL_SHIFT_SPEED"=w2302:u8, "READ_MODE"=w2301:u8, "VERTICAL_CLOCK_VOLTAGE"=w2300:u8, "AD_CHANNEL"=w2299:u32, "SHUTTER_MODE"=w2298:u8, "SHUTTER_TTL"=w2297:u8, "TRIGGER_MODE"=w2296:u8, "FRAME_TRANSFER"=w2295:bool, "ACQUISITION_MODE"=w2294:u8, "EM_MODE"=w2293:u8)
        n1056 = local read "Input Cluster"() -> (w2317:T5)
        n1057 = Bundle By Name(cluster=w2317, "Parameters.Image \nInitial Line"=w2313, "Parameters.Image\nInitial Column"=w2312, "Parameters.Image\nFinal Line"=w2311, "Parameters.Image\nFInal Column"=w2310, "Parameters.Vertical\nBinning"=w2309, "Parameters.Horizontal\nBinning"=w2308, "Parameters.Pre-amplification\nGain"=w2307, "Parameters.CCD\nEM Gain"=w2306, "Parameters.Readout\nRate"=w2305, "Parameters.Shutter\nOpenning Time"=w2304, "Parameters.Shutter\nClosing Time"=w2303, "Parameters.Vertical\nShift Speed"=w2302, "Parameters.Read\nMode"=w2301, "Parameters.Vertical\nClock Voltage"=w2300, "Parameters.A/D \nChannel"=w2299, "Parameters.Shutter\nMode"=w2298, "Parameters.Shutter\nTTL"=w2297, "Parameters.Trigger\nMode"=w2296, "Parameters.Frame\nTransfer"=w2295, "Parameters.Acquisition\nMode"=w2294, "Parameters.CCD \nEM Mode"=w2293) -> (w2316:T5)
        n1058 = local write "Input Cluster"(w2316) -> ()
      }
      event "Copy to Input ch4": Value Change {
        n1059 = event-data() -> ()  [unwired: 1 in, 6 out]
        n1060 = Unbundle By Name(w2328) -> ("Parameters"=w2327:T23)
        n1061 = Unbundle By Name(w2327) -> ("CCD \nEM Mode"=→"CCD \nEM Mode":u8)
        n1062 = property on="CCD \nEM Mode" class="DigNum (strict)" props=["Value"]() -> ()  [unwired: 2 in, 3 out]
        n1063 = call-dynamic "Read AcquisitionD.vi"("error in (no error)"=w2361, "S4ACS_GUI in"=w2362) -> ("error out"=w2357:errorcluster, "Acquisition.lvclass"=w2360:refnum<class "Acquisition.lvclass">, "S4ACS_GUI out"=w2329:refnum<class "S4GUI.lvclass">)  [unwired: 7 in]
        n1064 = call-dynamic "Read Channel.vi"("error in (no error)"=w2357, "Acquisition in"=w2360) -> ("error out"=w2356:errorcluster, "Channel.lvclass"=w2359:refnum<class "Channel.lvclass">)  [unwired: 7 in, 1 out]
        n1065 = call-dynamic "Read Interface.vi"("error in (no error)"=w2356, "Channel in"=w2359) -> ("error out"=w2355:errorcluster, "Interface.lvclass"=w2358:refnum<class "Interface.lvclass">)  [unwired: 7 in, 1 out]
        n1066 = call-dynamic "Get CCD_Config.vi"("error in (no error)"=w2355, "Interface in"=w2358) -> ("error out"=w2352:errorcluster, "output cluster"=w2351:T24)  [unwired: 7 in, 1 out]
        n1067 = Unbundle By Name(w2351) -> ("INITIAL_LINE"=w2350:u16, "INITIAL_COLUMN"=w2349:u16, "FINAL_LINE"=w2348:u16, "FINAL_COLUMN"=w2347:u16, "VBIN"=w2346:u16, "HBIN"=w2345:u16, "PREAMP"=w2344:u8, "EM_GAIN"=w2343:u16, "READOUT_RATE"=w2342:u8, "SHUTTER_OPENING_TIME"=w2341:u16, "SHUTTER_CLOSING_TIME"=w2340:u16, "VERTICAL_SHIFT_SPEED"=w2339:u8, "READ_MODE"=w2338:u8, "VERTICAL_CLOCK_VOLTAGE"=w2337:u8, "AD_CHANNEL"=w2336:u32, "SHUTTER_MODE"=w2335:u8, "SHUTTER_TTL"=w2334:u8, "TRIGGER_MODE"=w2333:u8, "FRAME_TRANSFER"=w2332:bool, "ACQUISITION_MODE"=w2331:u8, "EM_MODE"=w2330:u8)
        n1068 = local read "Input Cluster"() -> (w2354:T5)
        n1069 = Bundle By Name(cluster=w2354, "Parameters.Image \nInitial Line"=w2350, "Parameters.Image\nInitial Column"=w2349, "Parameters.Image\nFinal Line"=w2348, "Parameters.Image\nFInal Column"=w2347, "Parameters.Vertical\nBinning"=w2346, "Parameters.Horizontal\nBinning"=w2345, "Parameters.Pre-amplification\nGain"=w2344, "Parameters.CCD\nEM Gain"=w2343, "Parameters.Readout\nRate"=w2342, "Parameters.Shutter\nOpenning Time"=w2341, "Parameters.Shutter\nClosing Time"=w2340, "Parameters.Vertical\nShift Speed"=w2339, "Parameters.Read\nMode"=w2338, "Parameters.Vertical\nClock Voltage"=w2337, "Parameters.A/D \nChannel"=w2336, "Parameters.Shutter\nMode"=w2335, "Parameters.Shutter\nTTL"=w2334, "Parameters.Trigger\nMode"=w2333, "Parameters.Frame\nTransfer"=w2332, "Parameters.Acquisition\nMode"=w2331, "Parameters.CCD \nEM Mode"=w2330) -> (w2353:T5)
        n1070 = local write "Input Cluster"(w2353) -> ()
      }
      event "Scrollbar": Value Change {
        (unwired) 765.0 ("BarOffset")
        n1071 = event-data() -> ()  [unwired: 1 in, 6 out]
        n1072 = disable-structure shown="Disabled" {
          disable-tunnel: w2364 -> [w2376 _]
          frame Disabled {
            # "como alterar o valor de um parametro em \"Parameter Input\""
            n1073 = Unbundle By Name(w2376) -> ("Parameters"=w2378:T23)
            n1074 = Bundle By Name(cluster=w2378, "Readout\nRate"=u8 1 ("Readout\nRate")) -> (w2375:T23)
            n1075 = Bundle By Name(cluster=w2376, "Parameters"=w2375) -> (w2374:T5)
            n1076 = local write "Input Cluster"(w2374) -> ()
          }
          frame Enabled {
          }
        }
        n1077 = property on="Scrollbar" class="Scroll (strict)"() -> ("DocMax"=w2368:dbl)  [unwired: 2 in, 2 out]
        n1078 = Unbundle(w2366) -> ("Parameters"=w2371:refnum<vi>, "Current Configuration"=w2370:refnum<vi>)
        n1079 = Subtract(x=w2368, y="Scrollbar") -> (x-y=w2372:dbl)
        n1080 = Subtract(x=w2372, y=1000.0 ("BarOffset")) -> (x-y=w2369:dbl)
        n1081 = property on="Property Node" class="Clust (strict)"(reference=w2371, "Top"=w2369) -> ()  [unwired: 1 in, 2 out]
        n1082 = property on="Property Node" class="Clust (strict)"(reference=w2370, "Top"=w2369) -> ()  [unwired: 1 in, 2 out]
      }
      event "Select Positions": Value Change {
        # "Garantir que, quando em POLARIMETRIA, pelo menos WP1 esteja selecionado."
        n1083 = event-data() -> ()  [unwired: 1 in, 6 out]
        n1084 = call "Read Instrument.lvclass.vi"("error in (no error)"=w2400, "S4ACS_GUI in"=w2399) -> ("error out"=w2409:errorcluster, "Instrument.lvclass"=w2408:refnum<class "Instrument.lvclass">, "S4ACS_GUI out"=w2402:refnum<class "S4GUI.lvclass">)  [unwired: 7 in]
        n1085 = call "Read WPROT.vi"("error in (no error)"=w2409, "Instrument in"=w2408) -> ("error out"=w2401:errorcluster, "Opt_Selector.lvclass"=w2405:refnum<class "Opt_Selector.lvclass">, "Instrument out"=w2403:refnum<class "Instrument.lvclass">)  [unwired: 7 in]
        n1086 = case shown="4" "Select Positions" {
          tunnel: w2401 -> [w2443 w2456 w2469 w2482 w2495 w2504]
          tunnel: [w2441 w2454 w2467 w2477 w2493 w2503] -> w2404
          tunnel: [w2438 w2452 w2465 w2479 w2491 w2504] -> w2397
          tunnel: w2405 -> [w2444 w2457 w2470 w2483 w2496 w2503]
          tunnel: [16 8 4 8 0 0] -> w2398
          tunnel: [0.0 ("Scale.Range:Minimum") 0.0 ("Scale.Range:Minimum") 0.0 ("Scale.Range:Minimum") 0.0 ("Scale.Range:Minimum") 0.0 ("Scale.Range:Minimum") 0.0 ("Scale.Range:Minimum")] -> w2396
          frame 0, Default {
            w2440 = u16 65535 ("sequencia")
            w2445 = TRUE ("P0")
            w2446 = TRUE ("P0")
            w2447 = TRUE ("P0")
            w2448 = TRUE ("P0")
            # "1111 1111 1111 1111 = 65.535"
            n1087 = local write "P0"(w2448) -> ()
            n1088 = local write "P1"(w2448) -> ()
            n1089 = local write "P2"(w2448) -> ()
            n1090 = local write "P3"(w2448) -> ()
            n1091 = local write "P4"(w2446) -> ()
            n1092 = local write "P5"(w2446) -> ()
            n1093 = local write "P6"(w2446) -> ()
            n1094 = local write "P7"(w2446) -> ()
            n1095 = call-dynamic "Write sequencia.vi"("error in (no error)"=w2443, "sequencia"=w2440, "Opt_Selector in"=w2444) -> ("error out"=w2439:errorcluster, "Opt_Selector out"=w2442:refnum<class "Opt_Selector.lvclass">)  [unwired: 7 in]
